vi "sort.vi"() -> ()   [LabVIEW 2020]
uses:
  d1af0739-66d6-498a-b646-698bd5056a32.vi
  <vilib>/Comparison/Less/Less Functor/Less Functor.lvclass
panel:
  out "x-y 4":u32
  out "x-y 3":u32
  out "x-y 2":u32
  out "разница между самым быстрым и самым долгим методом":u32
  out "сортировка гномья в милисекундах":u32 caption="x-y"
  out "сортировка перемешиванием в милисекундах":u32 caption="x-y"
  out "сортировка вставкой в милисекундах":u32 caption="x-y"
  out "Boolean":bool
  out "Отср. массив гномья":i32[](array[numeric])
  out "Отср. массив перемещением":i32[](array[numeric])
  out "Отср. массив вставкой":i32[](array[numeric])
  out "Отср. массив 1D":i32[](array[numeric])
  out "Массив":i32[](array[numeric])
  in  "Кон. значение":dbl
  in  "Нач. значение":dbl
  in  "Кол-во":dbl
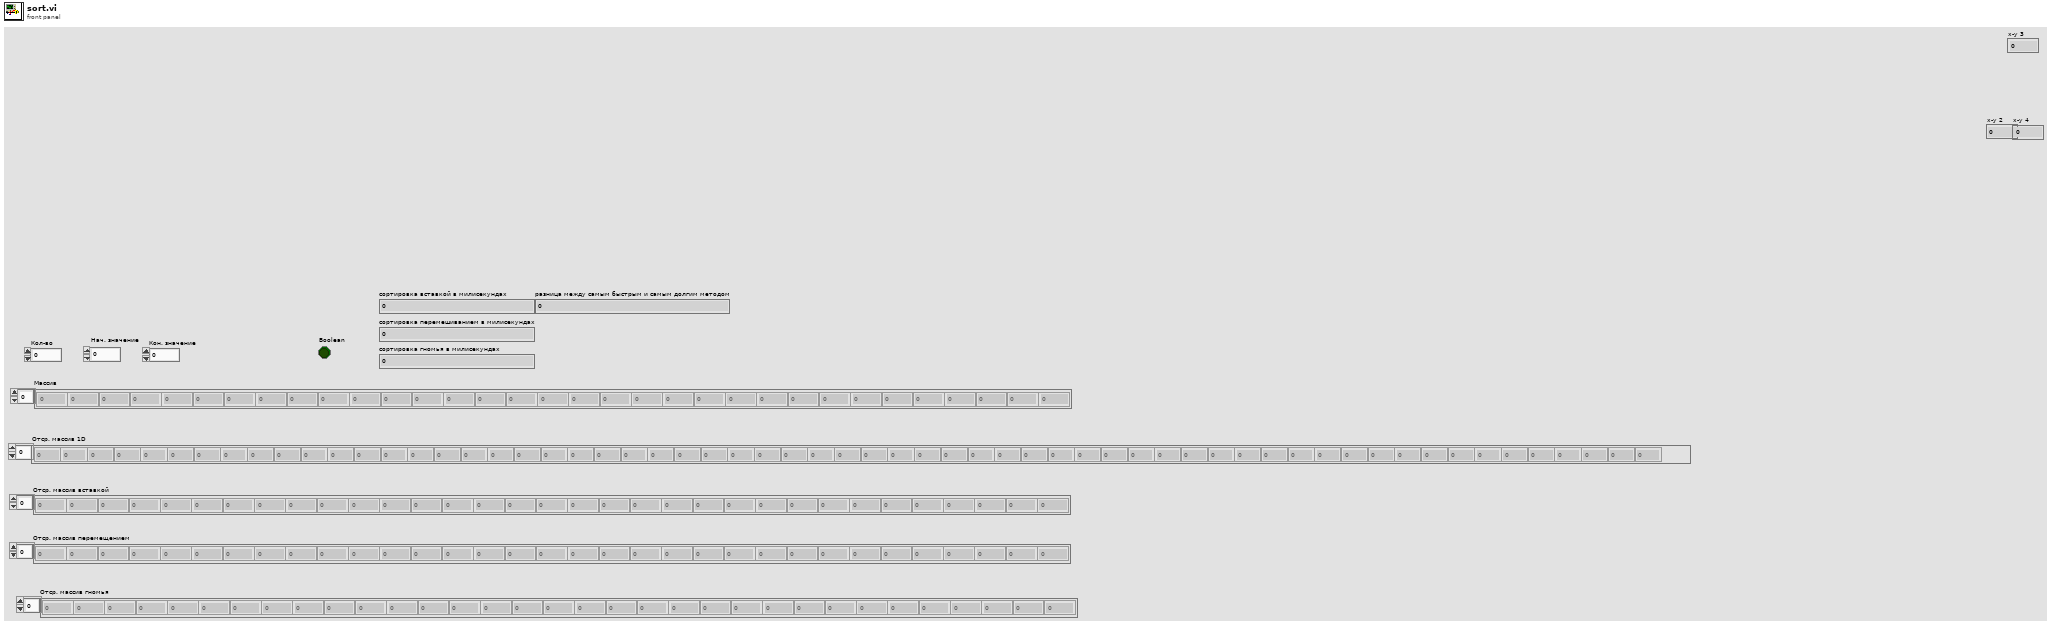
[diagram p1: front panel]
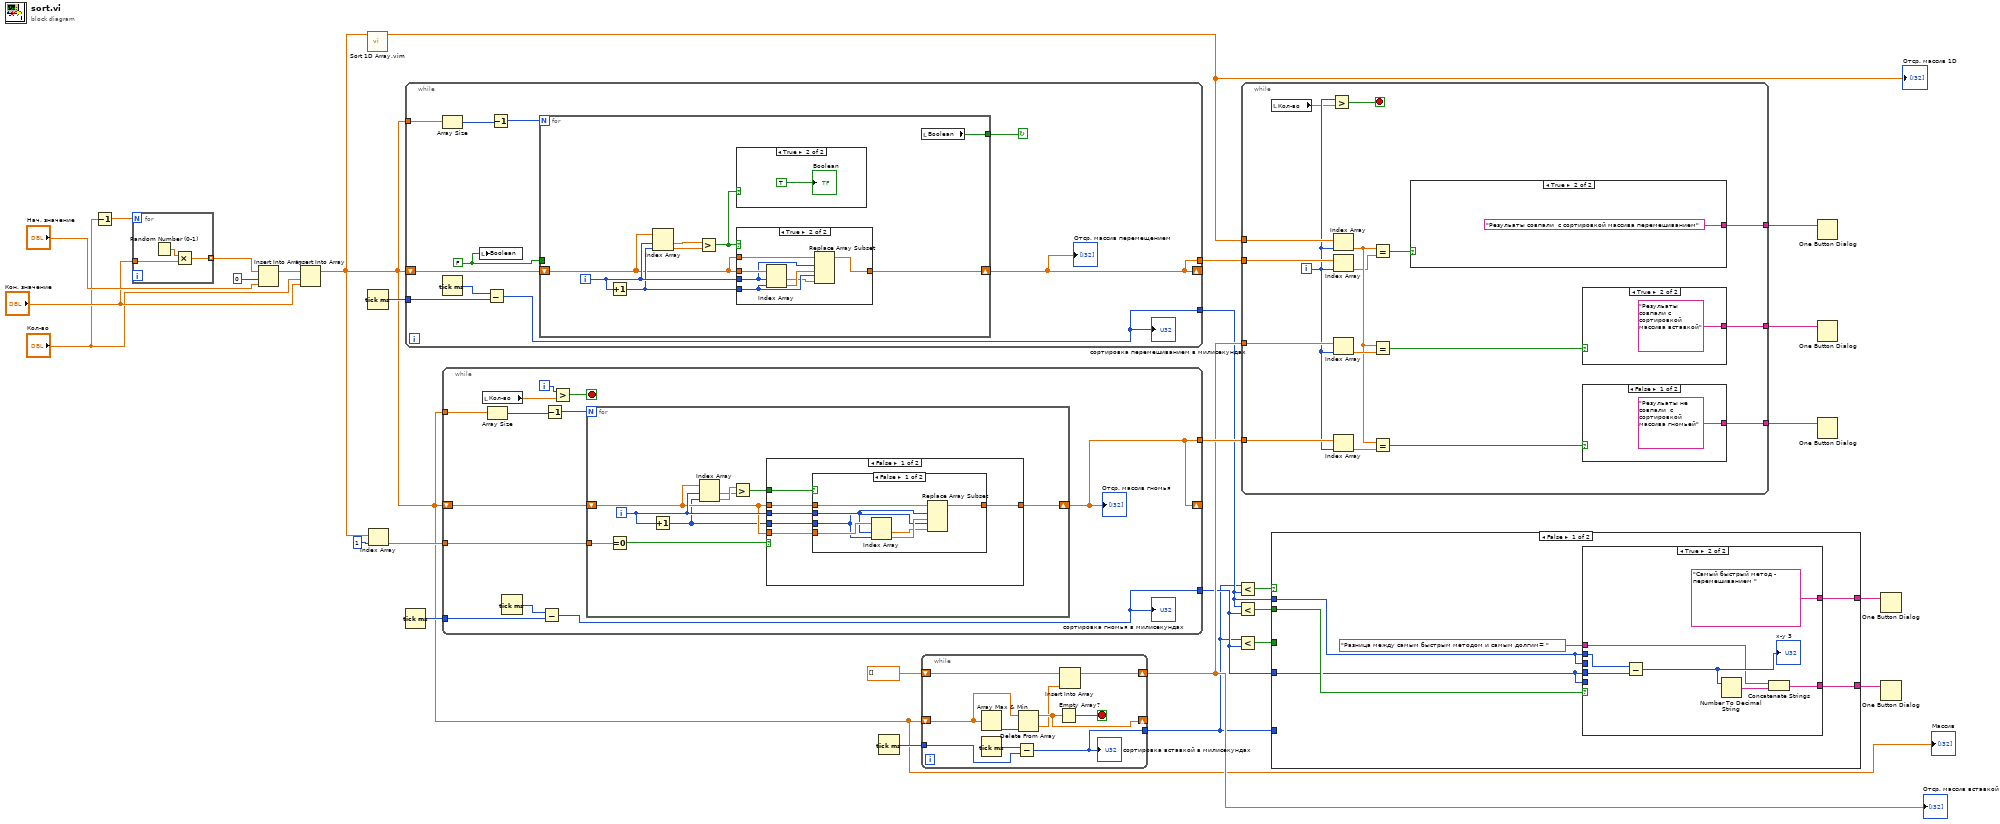
[diagram p0: block diagram]
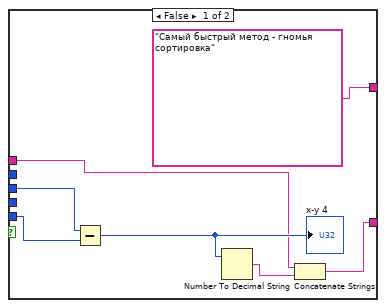
[diagram p2: hidden frame]
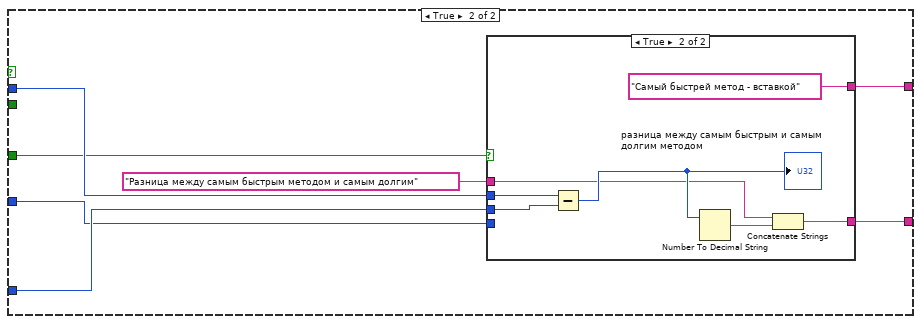
[diagram p3: hidden frame]
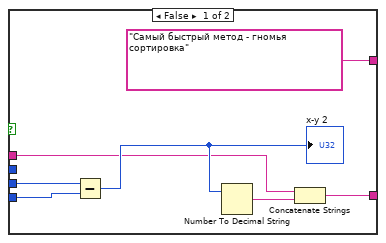
[diagram p4: hidden frame]
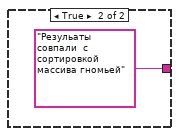
[diagram p5: hidden frame]
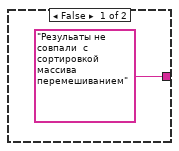
[diagram p6: hidden frame]
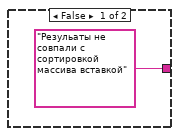
[diagram p7: hidden frame]
diagram:
  n1 = Decrement(x="Кол-во") -> (x-1=w1:dbl)
  n2 = for {
    N: w1 -> [_]
    tunnel: [w31] -> w27 mode=indexing
    tunnel: "Кон. значение" -> [w30]
    n3 = Random Number (0-1)() -> (number: 0 to 1=w32:dbl)
    n4 = Multiply(x=w32, y=w30) -> (x*y=w31:dbl)
  }
  n5 = Insert Into Array(array=w27, index=0, new element="Нач. значение") -> (w5:dbl[])
  n6 = Insert Into Array(array=w5, index="Кол-во", new element="Кон. значение") -> (w4:dbl[])
  "Массив" <- w4
  n7 = call "Sort 1D Array.vim"("unsorted array"=w4) -> ("sorted array"=w25:dbl[])  [unwired: 10 in]
  "Отср. массив 1D" <- w25
  n8 = Tick Count (ms)() -> (millisecond timer value=w17:u32)
  n9 = Index Array(array=w4, index=1) -> (element=w15:dbl)
  n10 = while {
    tunnel: w4 -> [w42]
    shift-right: [w36] -> _
    shift-left: w4 -> [w39]
    tunnel: [w36] -> w24
    tunnel: w17 -> [w34]
    tunnel: [w33] -> w7
    stop <- w37 continue-if-true
    w38 = FALSE
    n11 = Array Size(array=w42) -> (size(s)=w41:i32)
    n12 = Tick Count (ms)() -> (millisecond timer value=w35:u32)
    n13 = local write "Boolean"(w38) -> ()
    n14 = Subtract(x=w35, y=w34) -> (x-y=w33:u32)
    "сортировка перемешиванием в милисекундах" <- w33
    n15 = Decrement(x=w41) -> (x-1=w40:i32)
    n16 = for {
      N: w40 -> [_]
      shift-right: [w46] -> w36
      shift-left: w39 -> [w45]
      tunnel: w38 -> [_]
      tunnel: [w43] -> w37
      i -> [w48]
      n17 = Increment(x=w48) -> (x+1=w47:i32)
      n18 = Index Array(array=w45, index #1=w48, index #2=w47) -> (element #1=w50:dbl, element #2=w49:dbl)
      n19 = Greater?(x=w50, y=w49) -> (0:w44:bool)
      n20 = case shown="True" w44 {
        frame False {
        }
        frame True {
          "Boolean" <- TRUE
        }
      }
      n21 = case shown="True" w44 {
        tunnel: w48 -> [_ w58]
        tunnel: w47 -> [_ w57]
        tunnel: w45 -> [w52 w59]
        tunnel: [w52 w54] -> w46
        tunnel: w45 -> [_ w53]
        frame False {
        }
        frame True {
          n22 = Index Array(array=w59, index #1=w58, index #2=w57) -> (element #1=w55:dbl, element #2=w56:dbl)
          n23 = Replace Array Subset(array=w53, new element #1=w56, index #1=w58, new element #2=w55, index #2=w57) -> (w54:dbl[])
        }
      }
      n24 = local read "Boolean"() -> (w43:bool)
    }
    "Отср. массив перемещением" <- w36
  }
  n25 = Tick Count (ms)() -> (millisecond timer value=w18:u32)
  n26 = while {
    tunnel: w4 -> [w69]
    shift-right: [w64] -> _
    shift-left: w4 -> [w68]
    tunnel: [w64] -> w23
    tunnel: w18 -> [w62]
    tunnel: w15 -> [w61]
    tunnel: [w60] -> w8
    i -> [w65]
    stop <- w66 stop-if-true
    n27 = local read "Кол-во"() -> (w67:dbl)
    n28 = Array Size(array=w69) -> (size(s)=w71:i32)
    n29 = Tick Count (ms)() -> (millisecond timer value=w63:u32)
    n30 = Subtract(x=w63, y=w62) -> (x-y=w60:u32)
    "сортировка гномья в милисекундах" <- w60
    n31 = Decrement(x=w71) -> (x-1=w70:i32)
    n32 = Greater?(x=w65, y=w67) -> (0:w66:bool)
    n33 = for {
      N: w70 -> [_]
      shift-right: [w80] -> w64
      shift-left: w68 -> [w75]
      tunnel: w61 -> [w73]
      i -> [w76]
      n34 = Equal To 0?(x=w73) -> (x = 0?=w72:bool)
      n35 = Increment(x=w76) -> (x+1=w74:i32)
      n36 = Index Array(array=w75, index #1=w76, index #2=w74) -> (element #1=w77:dbl, element #2=w78:dbl)
      n37 = Greater?(x=w78, y=w77) -> (0:w79:bool)
      n38 = case shown="False" w72 {
        tunnel: [w85 w95] -> w80
        tunnel: w75 -> [w86 w95]
        tunnel: w79 -> [w84 _]
        tunnel: w76 -> [w83 _]
        tunnel: w75 -> [w82 _]
        tunnel: w74 -> [w81 _]
        frame False {
          n39 = case shown="False" w84 {
            tunnel: w86 -> [w90 w94]
            tunnel: [w91 w94] -> w85
            tunnel: w83 -> [w88 _]
            tunnel: w82 -> [w89 _]
            tunnel: w81 -> [w87 _]
            frame False {
              n40 = Index Array(array=w89, index #1=w88, index #2=w87) -> (element #1=w92:dbl, element #2=w93:dbl)
              n41 = Replace Array Subset(array=w90, new element #1=w93, index #1=w88, new element #2=w92, index #2=w87) -> (w91:dbl[])
            }
            frame True {
            }
          }
        }
        frame True {
        }
      }
    }
    "Отср. массив гномья" <- w64
  }
  n42 = Tick Count (ms)() -> (millisecond timer value=w16:u32)
  n43 = while {
    shift-right: [w103] -> _
    shift-left: w4 -> [w104]
    shift-right: [w100] -> w19
    shift-left: dbl[] [] -> [w101]
    tunnel: w16 -> [w97]
    tunnel: [w96] -> w6
    stop <- w105 stop-if-true
    n44 = Array Max & Min(array=w104) -> (min index (indices)=w102:i32)  [unwired: 3 out]
    n45 = Tick Count (ms)() -> (millisecond timer value=w98:u32)
    n46 = Subtract(x=w98, y=w97) -> (x-y=w96:u32)
    "сортировка вставкой в милисекундах" <- w96
    n47 = Delete From Array(array=w104, index=w102) -> (deleted portion=w99:dbl, array with subset deleted=w103:dbl[])  [unwired: 1 in]
    n48 = Empty Array?(array=w103) -> (empty?=w105:bool)
    n49 = Insert Into Array(array=w101, new element=w99) -> (w100:dbl[])  [unwired: 1 in]
  }
  "Отср. массив вставкой" <- w19
  n50 = Less?(x=w6, y=w7) -> (x < y?=w13:bool)
  n51 = Less?(x=w7, y=w8) -> (x < y?=w10:bool)
  n52 = Less?(x=w6, y=w8) -> (x < y?=w12:bool)
  n53 = while {
    tunnel: w25 -> [w122]
    tunnel: w19 -> [w121]
    tunnel: w24 -> [w118]
    tunnel: w23 -> [w117]
    tunnel: [w108] -> w21
    tunnel: [w107] -> w20
    tunnel: [w106] -> w22
    i -> [w111]
    stop <- w109 stop-if-true
    n54 = local read "Кол-во"() -> (w110:dbl)
    n55 = Greater?(x=w111, y=w110) -> (0:w109:bool)
    n56 = Index Array(array=w122, index=w111) -> (element=w116:dbl)
    n57 = Index Array(array=w118, index=w111) -> (element=w115:dbl)
    n58 = Index Array(array=w121, index=w111) -> (element=w120:dbl)
    n59 = Index Array(array=w117, index=w111) -> (element=w114:dbl)
    n60 = Equal?(x=w116, y=w115) -> (x = y?=w113:bool)
    n61 = Equal?(x=w116, y=w120) -> (x = y?=w119:bool)
    n62 = Equal?(x=w116, y=w114) -> (x = y?=w112:bool)
    n63 = case shown="True" w113 {
      tunnel: ["Резульаты не совпали  с сортировкой массива перемешиванием" "Резульаты совпали  с сортировкой массива перемешиванием"] -> w108
      frame False {
      }
      frame True {
      }
    }
    n64 = case shown="True" w119 {
      tunnel: ["Резульаты не совпали с сортировкой массива вставкой" "Резульаты совпали с сортировкой массива вставкой"] -> w107
      frame False {
      }
      frame True {
      }
    }
    n65 = case shown="False" w112 {
      tunnel: ["Резульаты не совпали  с сортировкой массива гномьей" "Резульаты совпали  с сортировкой массива гномьей"] -> w106
      frame False {
      }
      frame True {
      }
    }
  }
  n66 = case shown="False" w13 {
    tunnel: w6 -> [_ w155]
    tunnel: w7 -> [w132 w154]
    tunnel: w12 -> [_ w153]
    tunnel: [w133 w152] -> w11
    tunnel: w10 -> [w134 _]
    tunnel: [w130 w151] -> w9
    tunnel: w8 -> [w131 w150]
    frame False {
      n67 = case shown="True" w134 {
        tunnel: ["Самый быстрый метод - гномья сортировка" "Самый быстрый метод - перемешиванием "] -> w133
        tunnel: w132 -> [_ w146]
        tunnel: w131 -> [_ w145]
        tunnel: w132 -> [w139 _]
        tunnel: w131 -> [w138 _]
        tunnel: [w137 w142] -> w130
        tunnel: "Разница между самым быстрым методом и самым долгим= " -> [w136 w144]
        frame False {
          n68 = Subtract(x=w139, y=w138) -> (x-y=w140:u32)
          "x-y 4" <- w140
          n69 = Number To Decimal String(number=w140) -> (decimal integer string=w135:string)  [unwired: 1 in]
          n70 = Concatenate Strings(w136, w135) -> (w137:string)
        }
        frame True {
          n71 = Subtract(x=w146, y=w145) -> (x-y=w147:u32)
          "x-y 3" <- w147
          n72 = Number To Decimal String(number=w147) -> (decimal integer string=w143:string)  [unwired: 1 in]
          n73 = Concatenate Strings(w144, w143) -> (w142:string)
        }
      }
    }
    frame True {
      n74 = case shown="True" w153 {
        tunnel: w155 -> [w159 w167]
        tunnel: w154 -> [_ w166]
        tunnel: ["Самый быстрый метод - гномья сортировка" "Самый быстрей метод - вставкой"] -> w152
        tunnel: [w158 w165] -> w151
        tunnel: w150 -> [w160 _]
        tunnel: "Разница между самым быстрым методом и самым долгим" -> [w157 w164]
        frame False {
          n75 = Subtract(x=w159, y=w160) -> (x-y=w161:u32)
          "x-y 2" <- w161
          n76 = Number To Decimal String(number=w161) -> (decimal integer string=w156:string)  [unwired: 1 in]
          n77 = Concatenate Strings(w157, w156) -> (w158:string)
        }
        frame True {
          n78 = Subtract(x=w166, y=w167) -> (x-y=w168:u32)
          "разница между самым быстрым и самым долгим методом" <- w168
          n79 = Number To Decimal String(number=w168) -> (decimal integer string=w163:string)  [unwired: 1 in]
          n80 = Concatenate Strings(w164, w163) -> (w165:string)
        }
      }
    }
  }
  n81 = One Button Dialog(message=w21) -> ()  [unwired: 1 in, 1 out]
  n82 = One Button Dialog(message=w20) -> ()  [unwired: 1 in, 1 out]
  n83 = One Button Dialog(message=w22) -> ()  [unwired: 1 in, 1 out]
  n84 = One Button Dialog(message=w11) -> ()  [unwired: 1 in, 1 out]
  n85 = One Button Dialog(message=w9) -> ()  [unwired: 1 in, 1 out]
